vi "MAXTdll.vi"(8 "error in (no error)":errorcluster, 11 "z":dbl[](array[numeric])) -> (0 "error out":errorcluster, 3 "Outputs":T1)   [LabVIEW 2015]
doc: "subroutine MAXTdll(z, tm, pm, dm, ierr, herr, herr_length)\n\nCalculate values at the maximum temperature along the saturation line; these are returned from the call to\nSATSPLN and apply only to the composition in the z() array sent to SATSPLN.\n\nINPUTS:\nz -- Composition (array of mole fractions)\n\nOUTPUTS:\ntm -- Temperature [K]\npm -- Pressure [kPa]\ndm -- Density [mol/L]\nierr -- Error flag: 0 - Successful, 331 - Splines not available for calculation 361 - Maximum temperature not known\nherr -- Error string (character*255)\nherr_length -- length of variable herr (default: 255)"
uses:
  REFPROP.dll
panel:
  # "REFPROP-MAXTdll.vi"
  # "void  MAXTdll(double *z, double *tm, double *pm, double *dm, int32_t *ierr, CStr herr, int32_t herr_length)"
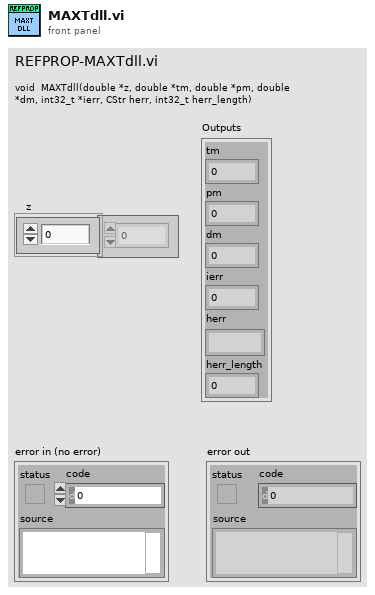
[diagram p1: front panel]
types:
  T1 = cluster{"tm":dbl, "pm":dbl, "dm":dbl, "ierr":i32, "herr":string, "herr_length":i32}
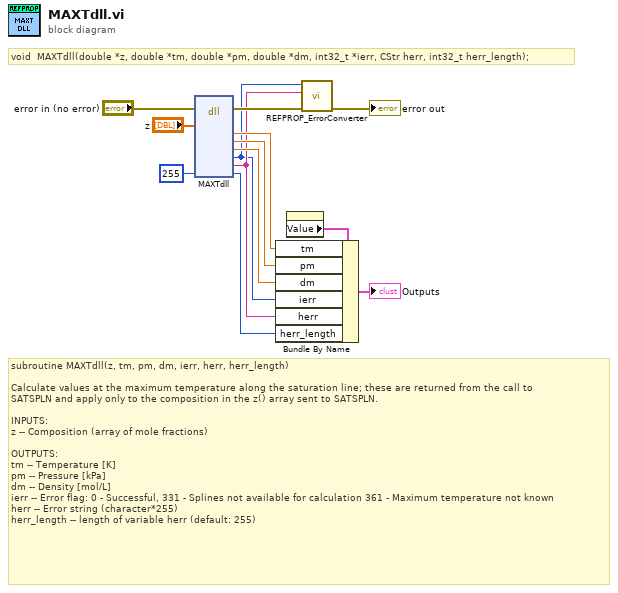
[diagram p0: block diagram]
diagram:
  # "void  MAXTdll(double *z, double *tm, double *pm, double *dm, int32_t *ierr, CStr herr, int32_t herr_length);"
  # "subroutine MAXTdll(z, tm, pm, dm, ierr, herr, herr_length)\n\nCalculate values at the maximum temperature along the saturation line; these are returned from the call to\nSATSPLN and apply only to the composition in the z() array sent to SATSPLN.\n\nINPUTS:\nz -- Composition (array of mole fractions)\n\nOUTPUTS:\ntm -- Temperature [K]\npm -- Pressure [kPa]\ndm -- Density [mol/L]\nierr -- Error flag: 0 - Successful, 331 - Splines not available for calculation 361 - Maximum temperature not known\nherr -- Error string (character*255)\nherr_length -- length of variable herr (default: 255)"
  n1 = dll-call lib="C:/Users/lauria/Desktop/REFPROP 10 LabVIEW Wrapper BETA/REFPROP/REFPROP.*" fn="MAXTdll"(error in="error in (no error)", "z"="z", "herr_length"=255 ("ln")) -> (error out=w11:errorcluster, "tm"=w3:dbl, "pm"=w4:dbl, "dm"=w5:dbl, "ierr"=w1:i32, "herr"=w2:string, "herr_length"=w6:i32)  [unwired: 9 in, 1 out]
  n2 = property on="Outputs" class="Clust (strict)"() -> ("Value"=w8:T1)  [unwired: 2 in, 2 out]
  n3 = Bundle By Name(cluster=w8, "tm"=w3, "pm"=w4, "dm"=w5, "ierr"=w1, "herr"=w2, "herr_length"=w6) -> (→"Outputs":T1)
  n4 = call "REFPROP_ErrorConverter.vi"("error in (no error)"=w11, "Error Message"=w2, "Error Code"=w1) -> ("error out"=→"error out":errorcluster)  [unwired: 8 in]
